vi "VG-GUI.vi"(8 "error in (no error)":errorcluster, 11 "VG-VNA_GUI in":refnum<class "VG-VNA_GUI.lvclass">) -> (0 "error out":errorcluster, 3 "VG-VNA_GUI out":refnum<class "VG-VNA_GUI.lvclass">)   [LabVIEW 2020, in "VG-VNA_GUI.lvlib" / "VG-VNA_GUI.lvclass"]
uses:
  VG-VNA_GUI.lvclass
  classes/vna-drivers/liteVNA/VD-settingsEasy.ctl
  classes/vna-drivers/liteVNA/VD-sampleSize.ctl
  C:/Program Files (x86)/National Instruments/LabVIEW 2020/vi.lib/ActorFramework/Actor/Actor.lvclass
  classes/vna-drivers/liteVNA/VD-connection_settings.ctl
  classes/hardware-protocol/serial/HP-S-baudrate.ctl
  classes/vna-drivers/liteVNA/VD-settings_status.ctl
  VG-VNA_GUI.lvclass/VG-VNA_GUI.ctl
  <vilib>/ActorFramework/Message Enqueuer/Message Enqueuer.lvclass/Message Enqueuer.ctl
  hardware_manager/VHM-VNA_Hardware_Manager/VHM-VNA_Hardware_Manager Messages/VHM-setSettings Msg/VHM-setSettings Msg.lvclass/VHM-setSettings Msg.ctl
  hardware_manager/VHM-VNA_Hardware_Manager/VHM-VNA_Hardware_Manager Messages/VHM-connectionSettings Msg/VHM-connectionSettings Msg.lvclass/VHM-connectionSettings Msg.ctl
  <vilib>/ActorFramework/Actor/Actor.lvclass/Actor.ctl
  <vilib>/ActorFramework/Message Enqueuer/Enqueue.vi
  <vilib>/ActorFramework/Message Enqueuer/Init from Existing Queue.vi
  hardware_manager/VHM-VNA_Hardware_Manager/VHM-VNA_Hardware_Manager Messages/VHM-connect Msg/VHM-connect Msg.lvclass
  C:/Program Files (x86)/National Instruments/LabVIEW 2020/vi.lib/ActorFramework/Message/Message.lvclass
  hardware_manager/VHM-VNA_Hardware_Manager/VHM-VNA_Hardware_Manager Messages/VHM-getDataSet Msg/VHM-getDataSet Msg.lvclass
  hardware_manager/VHM-VNA_Hardware_Manager/VHM-VNA_Hardware_Manager Messages/VHM-disconnect Msg/VHM-disconnect Msg.lvclass
  hardware_manager/VHM-VNA_Hardware_Manager/VHM-VNA_Hardware_Manager Messages/VHM-setSettings Msg/VHM-setSettings Msg.lvclass
  hardware_manager/VHM-VNA_Hardware_Manager/VHM-VNA_Hardware_Manager Messages/VHM-connectionSettings Msg/VHM-connectionSettings Msg.lvclass
  <vilib>/ActorFramework/Stop Msg/Stop Msg.lvclass
  <vilib>/ActorFramework/Message Priority Queue/Priority Enqueue.vi
  <vilib>/ActorFramework/Message Enqueuer/Message Enqueuer.lvclass
  <vilib>/ActorFramework/Actor/Actor.lvclass
  classes/vna-drivers/liteVNA/VD-LV-LiteVNA.lvclass
  classes/hardware-protocol/serial/HP-S-Serial.lvclass
panel:
  in  "settings":T1={"Start [hz]"=1000000, "Stop [hz]"=5000000, "sampleSize"=101} {"sampleSize" items=["101"=101, "201"=201, "401"=401, "601"=601, "801"=801, "1001"=1001]; "Stop [hz]" format="%.0p"; "Start [hz]" format="%.0p"}
  in  "Set Settings":bool
  in  "connection settings":T3={"Com"="", "baud rate (9600)"=38400} {"baud rate (9600)" items=["75"=75, "110"=110, "134"=134, "150"=150, "300"=300, "600"=600, "1200"=1200, "1800"=1800, "2400"=2400, "4800"=4800, "7200"=7200, "9600"=9600, "14400"=14400, "19200"=19200, "28800"=28800, "38400"=38400, "56000"=56000, "57600"=57600, "115200"=115200, "128000"=128000, "230400"=230400]}
  in  "Connect":bool
  in  "Disconnect":bool
  in  "Set connection settings":bool
  out "Settings status":T5
  in  "Tab Control":enum32{"Graph", "Other"}(tab)
  out "XY Graph 2":cluster{u64[], dbl[]}[](graph)
  out "XY Graph":cluster{u64[], dbl[]}[](graph)
  in  "get set":bool
  in  "Stop":bool
  out "error IO":errorcluster
  out "Last change":timestamp
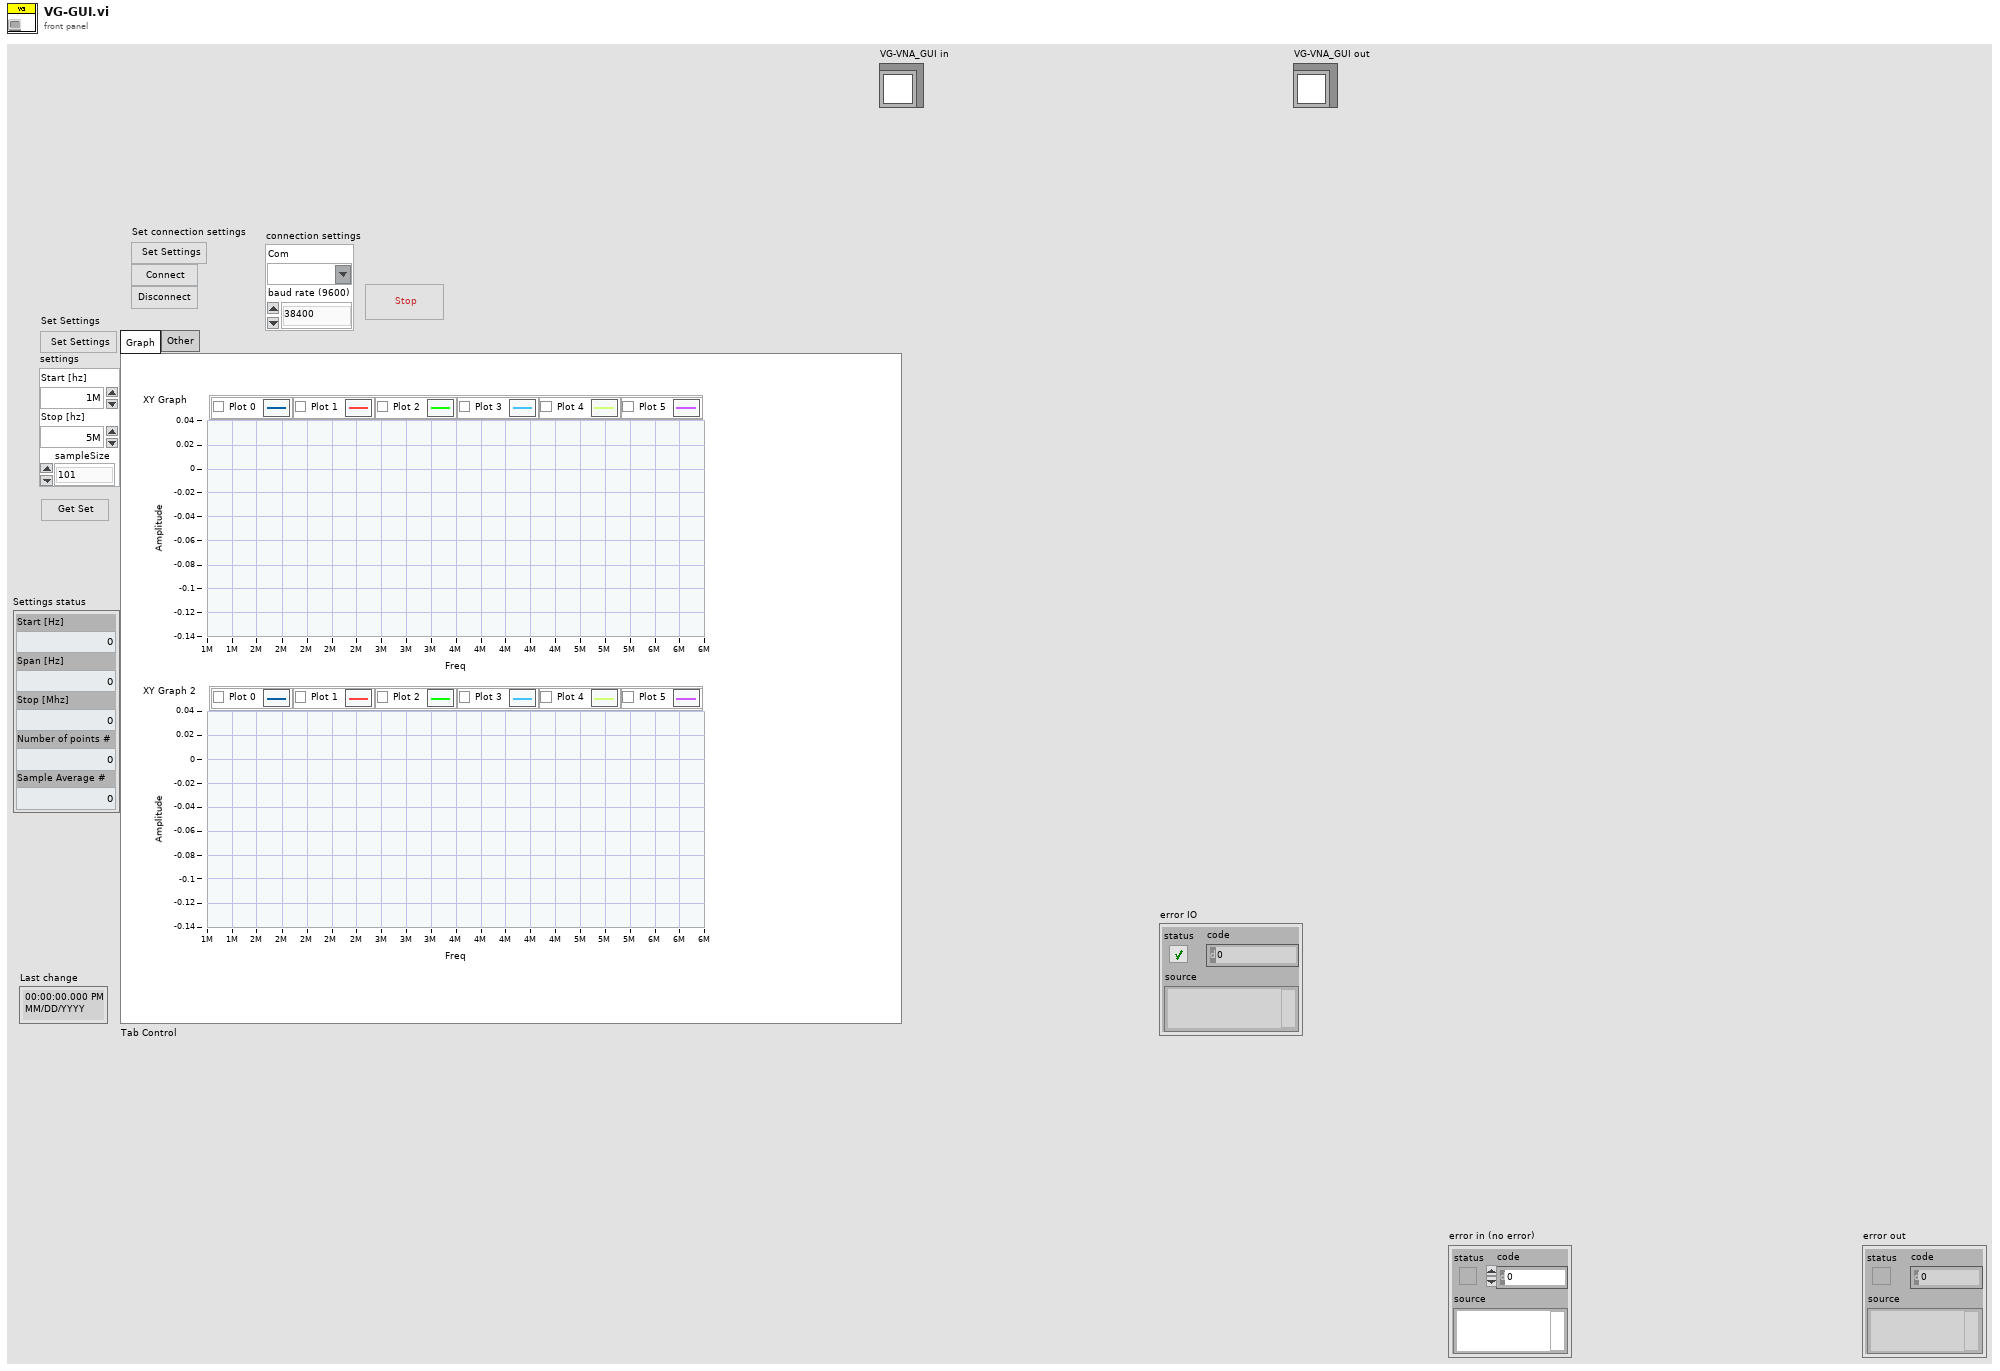
[diagram p1: front panel]
types:
  T1 = typedef "VD-LV-LiteVNA.lvclass/VD-settingsEasy.ctl" = cluster{"Start [hz]":u64, "Stop [hz]":u64, "sampleSize":T2}
  T2 = typedef "VD-LV-LiteVNA.lvclass/VD-sampleSize.ctl" = u16
  T3 = typedef "VD-LV-LiteVNA.lvclass/VD-connection_settings.ctl" = cluster{"Com":refnum<visa-resource-name>, "baud rate (9600)":T4}
  T4 = typedef "HP-S-Serial.lvclass/HP-S-baudrate.ctl" = u32
  T5 = typedef "VD-LV-LiteVNA.lvclass/VD-settings_status.ctl" = cluster{"Start [Hz]":u64, "Span [Hz]":u64, "Stop [Mhz]":u64, "Number of points #":u16, "Sample Average #":u16}
  T6 = cluster{"Stop":refnum<user-event>, "Graph Data":refnum<user-event>, "Settings status":refnum<user-event>, "Calibration Status":refnum<user-event>, "connection status":refnum<user-event>}
  T7 = typedef "VG-VNA_GUI.lvlib/VG-VNA_GUI.lvclass/VG-graph_data.ctl" = cluster{u64[], dbl[]}[]
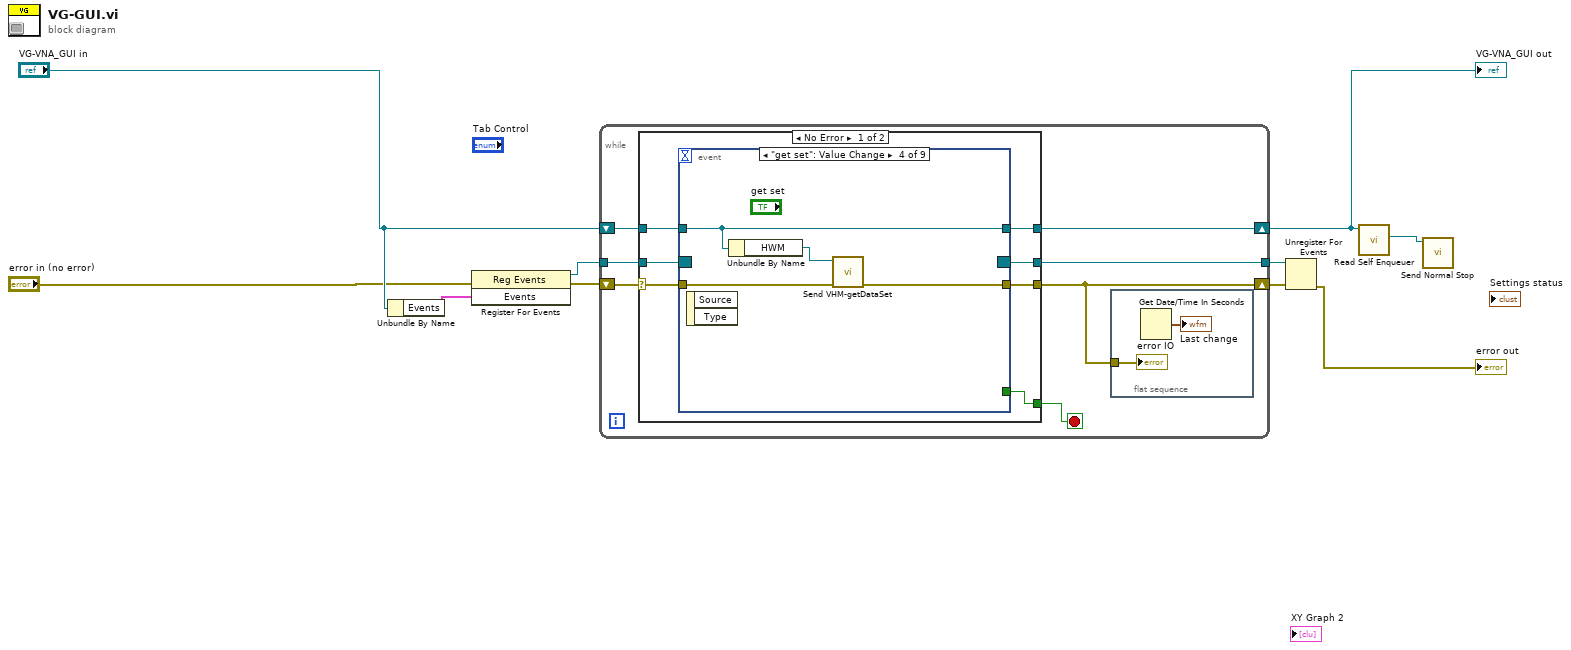
[diagram p0: block diagram]
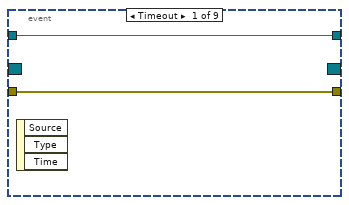
[diagram p2: hidden frame]
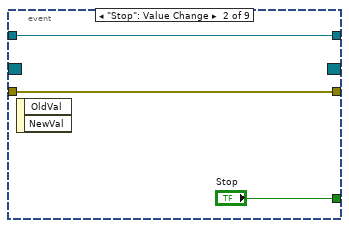
[diagram p3: hidden frame]
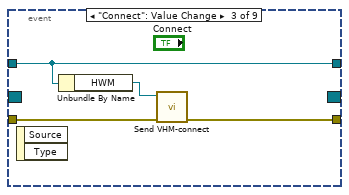
[diagram p4: hidden frame]
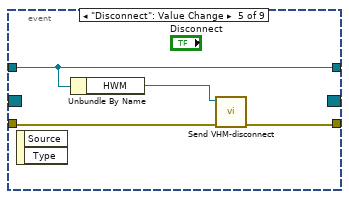
[diagram p5: hidden frame]
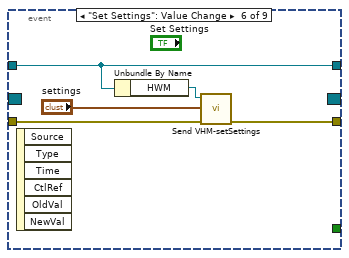
[diagram p6: hidden frame]
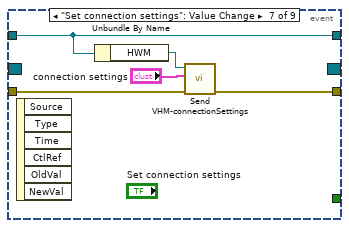
[diagram p7: hidden frame]
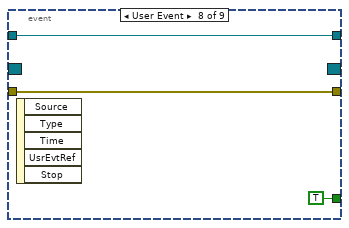
[diagram p8: hidden frame]
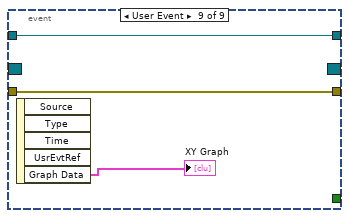
[diagram p9: hidden frame]
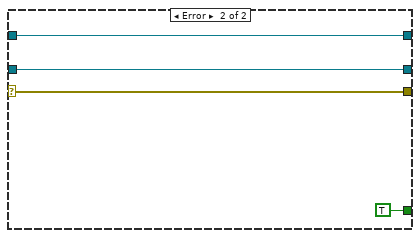
[diagram p10: hidden frame]
diagram:
  n1 = Unbundle By Name("VG-VNA_GUI in") -> ("Events"=w6:T6)
  n2 = register-events(error in="error in (no error)", w6) -> (reference out=w5:refnum<event-registration>, error out=w7:errorcluster)  [unwired: 1 in]
  n3 = while {
    shift-right: [w15] -> w9
    shift-left: w7 -> [w16]
    shift-right: [w13] -> w1
    shift-left: "VG-VNA_GUI in" -> [w14]
    tunnel: [w12] -> w8
    tunnel: w5 -> [w11]
    stop <- w17 stop-if-true
    n4 = case shown="No Error" w16 {
      selector: w16 -> [w26 w62]
      tunnel: [w24 TRUE] -> w17
      tunnel: [w25 w62] -> w15
      tunnel: w14 -> [w23 w61]
      tunnel: [w22 w61] -> w13
      tunnel: [w21 w60] -> w12
      tunnel: w11 -> [w20 w60]
      frame No Error {
        n5 = event shown="[3] \"get set\": Value Change" {
          selector: w20 -> [_ _ _ _ _ _ _ _ _]
          dyn-events: [_ _ _ _ _ _ _ _ _] -> w21
          timeout: _ -> [_ _ _ _ _ _ _ _ _]
          tunnel: w26 -> [w28 w30 w35 w38 w42 w48 w50 w56 w59]
          tunnel: [w28 w30 w34 w36 w40 w47 w49 w56 w59] -> w25
          tunnel: [_ "Stop" _ _ _ _ _ TRUE ("Stop") _] -> w24
          tunnel: w23 -> [w27 w29 w32 w39 w43 w45 w53 w55 w58]
          tunnel: [w27 w29 w32 w39 w43 w45 w53 w55 w58] -> w22
          event Timeout {
            n6 = event-data() -> ()  [unwired: 1 in, 3 out]
          }
          event "Stop": Value Change {
            n7 = event-data() -> ()  [unwired: 1 in, 2 out]
          }
          event "Connect": Value Change {
            n8 = event-data() -> ()  [unwired: 1 in, 2 out]
            n9 = Unbundle By Name(w32) -> ("HWM"=w33:refnum<class "Message Enqueuer.lvclass">)
            n10 = call "Send VHM-connect.vi"("error in (no error)"=w35, "Message Enqueuer"=w33) -> ("error out"=w34:errorcluster)  [unwired: 8 in, 1 out]
          }
          event "get set": Value Change {
            n11 = event-data() -> ()  [unwired: 1 in, 2 out]
            n12 = Unbundle By Name(w39) -> ("HWM"=w37:refnum<class "Message Enqueuer.lvclass">)
            n13 = call "Send VHM-getDataSet.vi"("error in (no error)"=w38, "Message Enqueuer"=w37) -> ("error out"=w36:errorcluster)  [unwired: 8 in, 1 out]
          }
          event "Disconnect": Value Change {
            n14 = event-data() -> ()  [unwired: 1 in, 2 out]
            n15 = Unbundle By Name(w43) -> ("HWM"=w41:refnum<class "Message Enqueuer.lvclass">)
            n16 = call "Send VHM-disconnect.vi"("error in (no error)"=w42, "Message Enqueuer"=w41) -> ("error out"=w40:errorcluster)  [unwired: 8 in, 1 out]
          }
          event "Set Settings": Value Change {
            n17 = event-data() -> ()  [unwired: 1 in, 6 out]
            n18 = Unbundle By Name(w45) -> ("HWM"=w44:refnum<class "Message Enqueuer.lvclass">)
            n19 = call "Send VHM-setSettings.vi"("error in (no error)"=w48, "settings"="settings", "Message Enqueuer"=w44) -> ("error out"=w47:errorcluster)  [unwired: 7 in, 1 out]
          }
          event "Set connection settings": Value Change {
            n20 = event-data() -> ()  [unwired: 1 in, 6 out]
            n21 = Unbundle By Name(w53) -> ("HWM"=w52:refnum<class "Message Enqueuer.lvclass">)
            n22 = call "Send VHM-connectionSettings.vi"("error in (no error)"=w50, "connection settings"="connection settings", "Message Enqueuer"=w52) -> ("error out"=w49:errorcluster)  [unwired: 7 in, 1 out]
          }
          event User Event {
            n23 = event-data() -> ()  [unwired: 1 in, 5 out]
          }
          event User Event {
            n24 = event-data() -> ("Graph Data"=→"XY Graph":T7)  [unwired: 1 in, 4 out]
          }
        }
      }
      frame Error {
      }
    }
    n25 = flat-sequence {
      tunnel: w15 -> [w19]
      frame #0 {
        n26 = Get Date/Time In Seconds() -> (seconds since 1Jan1904=→"Last change":timestamp)
        "error IO" <- w19
      }
    }
  }
  "VG-VNA_GUI out" <- w1
  n27 = Unregister For Events(event registration refnum=w8, error in=w9) -> (error out=→"error out":errorcluster)
  n28 = call <vilib>:"Read Self Enqueuer.vi"("Actor"=w1) -> ("Self Enqueuer"=w10:refnum<class "Message Enqueuer.lvclass">)  [unwired: 10 in]
  n29 = call <vilib>:"Send Normal Stop.vi"("Message Enqueuer"=w10) -> ()  [unwired: 10 in, 1 out]
